vi "CRC.vi"(0 "输入字符串":string) -> (1 "CRC高8位":u8 format="%x", 2 "CRC低8位":u8 format="%x")   [LabVIEW 2015]
panel:
  # "02030001000C"
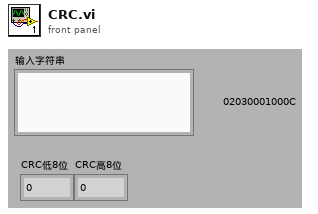
[diagram p1: front panel]
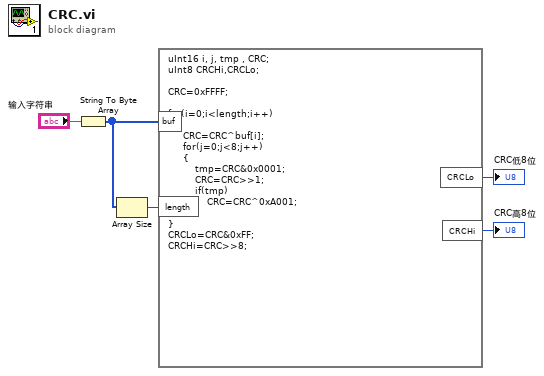
[diagram p0: block diagram]
diagram:
  n1 = String To Byte Array(string="输入字符串") -> (unsigned byte array=w3:u8[])
  n2 = Array Size(array=w3) -> (size(s)=w2:i32)
  n3 = formula code="uInt16 i, j, tmp , CRC;\nuInt8 CRCHi,CRCLo;\n\nCRC=0xFFFF;\n\nfor(i=0;i<length;i++)\n{\n     CRC=CRC^buf[i];\n     for(j=0;j<8;j++)\n     {\n         tmp=CRC&0x0001;\n         CRC=CRC>>1;\n         if(tmp)\n             CRC=CRC^0xA001;           \n     }\n}\nCRCLo=CRC&0xFF;\nCRCHi=CRC>>8;"("buf"=w3, "length"=w2) -> ("CRCLo"=→"CRC低8位":u8, "CRCHi"=→"CRC高8位":u8)
